vi "SDO_Trajectory_BEGIN.vi"(10 "gyroAngle":T1={"VALUE"=0.0, "COS"=1.0, "SIN"=0.0} {"SIN" format="%13.4f"; "COS" format="%13.4f"; "VALUE" format="%13.4f"}) -> ()   [LabVIEW 2019]
uses:
  <vilib>/Rock Robotics/WPI/ThirdParty/JAS_Junk/TrajLib/Trajectory_Library.lvlib
  SWERVE_TRAJECTORY_GLOBALS.vi
  <vilib>/Rock Robotics/WPI/ThirdParty/JAS_Junk/TrajLib/TypeDef/ROTATION2D.ctl
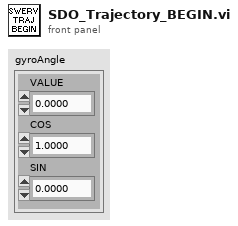
[diagram p1: front panel]
types:
  T1 = typedef "Trajectory_Library.lvlib/ROTATION2D.ctl" = cluster{"VALUE":dbl, "COS":dbl, "SIN":dbl}
  T2 = typedef "Trajectory_Library.lvlib/TRAJECTORY.ctl" = cluster{"TotalTImeSecs":dbl, "States":T3[]}
  T3 = typedef "Trajectory_Library.lvlib/TRAJ_STATE.ctl" = cluster{"TimeSeconds":dbl, "Velocity":dbl, "Acceleration":dbl, "POSE":T4, "Curvature":dbl}
  T4 = typedef "Trajectory_Library.lvlib/POSE2D.ctl" = cluster{"TRANSLATION":T5, "ROTATION":T1}
  T5 = typedef "Trajectory_Library.lvlib/TRANSLATION2D.ctl" = cluster{"X":dbl, "Y":dbl}
  T6 = typedef "Trajectory_Library.lvlib/SWERVE_DRIVE_MODULE_POSITION.ctl" = cluster{"Distance":dbl, "Angle":T1, "P":bool}
  T7 = typedef "Trajectory_Library.lvlib/SWERVE_DRIVE_ODOMETRY.ctl" = cluster{"POSE":T4, "GyroOffset":T1, "PreviousAngle":T1, "PrevModulePositions":T6[], "NumModules":i32}
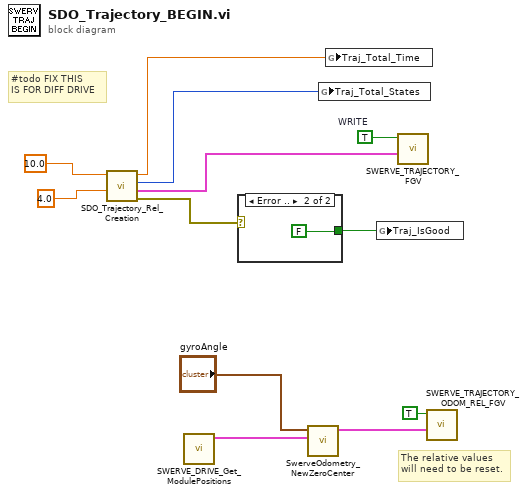
[diagram p0: block diagram]
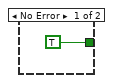
[diagram p2: hidden frame]
diagram:
  w7 = TRUE  # WRITE
  # "#todo FIX THIS\nIS FOR DIFF DRIVE"
  # "The relative values\nwill need to be reset."
  n1 = call "SDO_Trajectory_Rel_Creation.vi"("Effective Track Width Ft"=4.0, "Max Velocity Ft/Sec"=10.0) -> ("Trajectory  creation error"=w5:errorcluster, "Relative Trajectory"=w6:T2, "Trajectory Items"=w3:i32, "TotalTImeSecs"=w4:dbl)  [unwired: 6 in]
  n2 = call "SWERVE_DRIVE_Get_ModulePositions.vi"() -> ("Swerve Module Positions"=w8:T6[])  [unwired: 11 in]
  n3 = case shown="Error .." w5 {
    tunnel: [TRUE FALSE] -> w9
    frame No Error {
    }
    frame Error {
    }
  }
  n4 = call <vilib>:"SwerveOdometry_NewZeroCenter.vi"("Module Positions"=w8, "gyroAngle"="gyroAngle") -> ("SWERVE_DRIVE_ODOMETRY"=w12:T7)  [unwired: 9 in]
  n5 = global write "SWERVE_TRAJECTORY_GLOBALS.vi" "Traj_Total_States"(w3) -> ()
  n6 = global write "SWERVE_TRAJECTORY_GLOBALS.vi" "Traj_Total_Time"(w4) -> ()
  n7 = global write "SWERVE_TRAJECTORY_GLOBALS.vi" "Traj_IsGood"(w9) -> ()
  n8 = call "SWERVE_TRAJECTORY_FGV.vi"("inTRAJECTORY"=w6, "WRITE"=w7) -> ()  [unwired: 9 in, 1 out]
  n9 = call "SWERVE_TRAJECTORY_ODOM_REL_FGV.vi"("in SWERVE_DRIVE_ODOMETRY"=w12, "WRITE"=TRUE) -> ()  [unwired: 9 in, 1 out]
